vi "绑定设备.vi"(8 "error in (no error)":errorcluster, 10 "设备注册-来自PC总客户端":T1, 11 "数据库操作.i":refnum<class "数据库操作.lvclass">) -> (0 "error out":errorcluster, 3 "数据库操作.o":refnum<class "数据库操作.lvclass">)   [LabVIEW 2013, in "数据库操作.lvclass"]
uses:
  <vilib>/addons/database/Connection.llb/Conn Execute.vi
  <vilib>/addons/database/NI_Database_API.lvlib
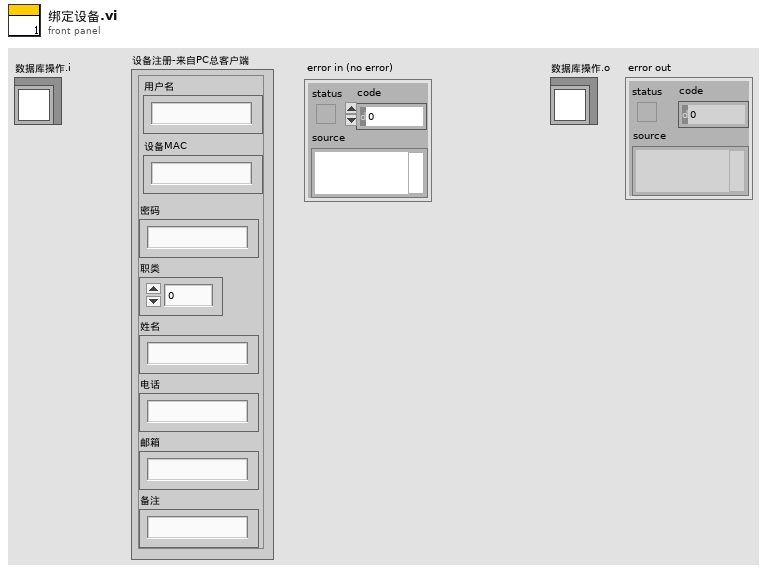
[diagram p1: front panel]
types:
  T1 = cluster{"设备MAC":string, "密码":string, "职类":i32, "姓名":string, "电话":string, "邮箱":string, "备注":string, "用户名":string}
  T2 = typedef "NI_Database_API.lvlib/Conn ObjectReference.ctl" = refnum<k1>
  T3 = cluster{"用户名":string, "设备状态":i32, "密码":string, "职类":i32, "姓名":string, "电话":string, "邮箱":string, "备注":string, "最后活动":string}
  T4 = enum16{"用户名", "设备MAC", "设备状态", "密码", "职类", "姓名", "电话", "邮箱", "备注", "最后活动"}
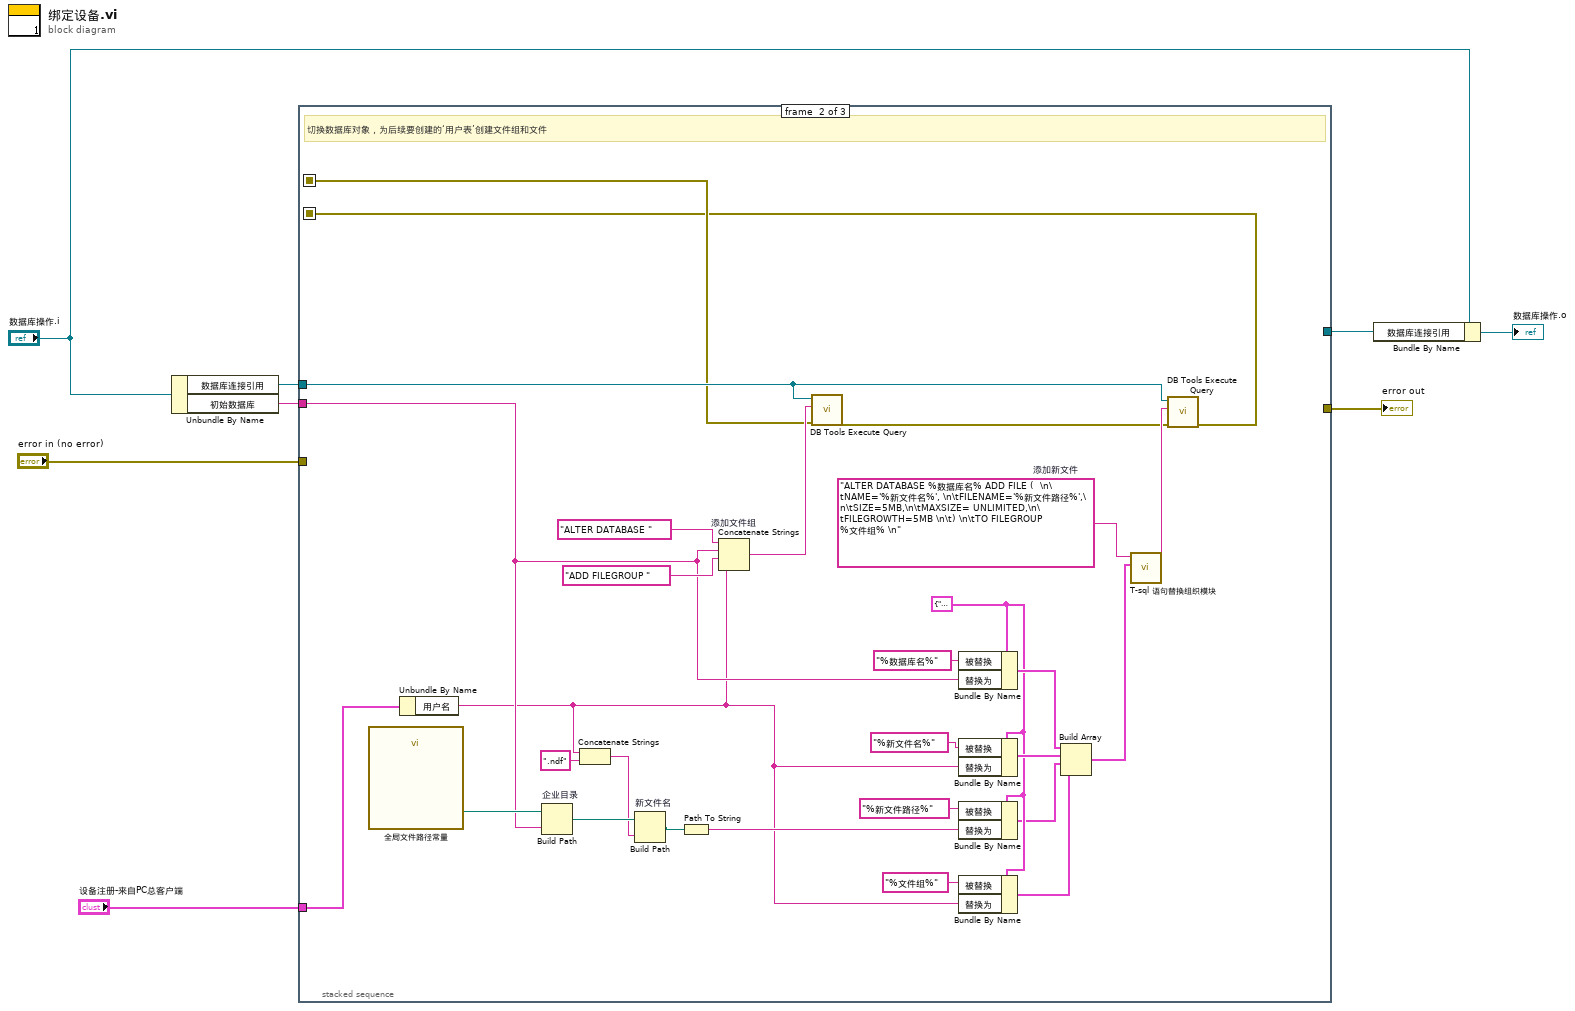
[diagram p0: block diagram]
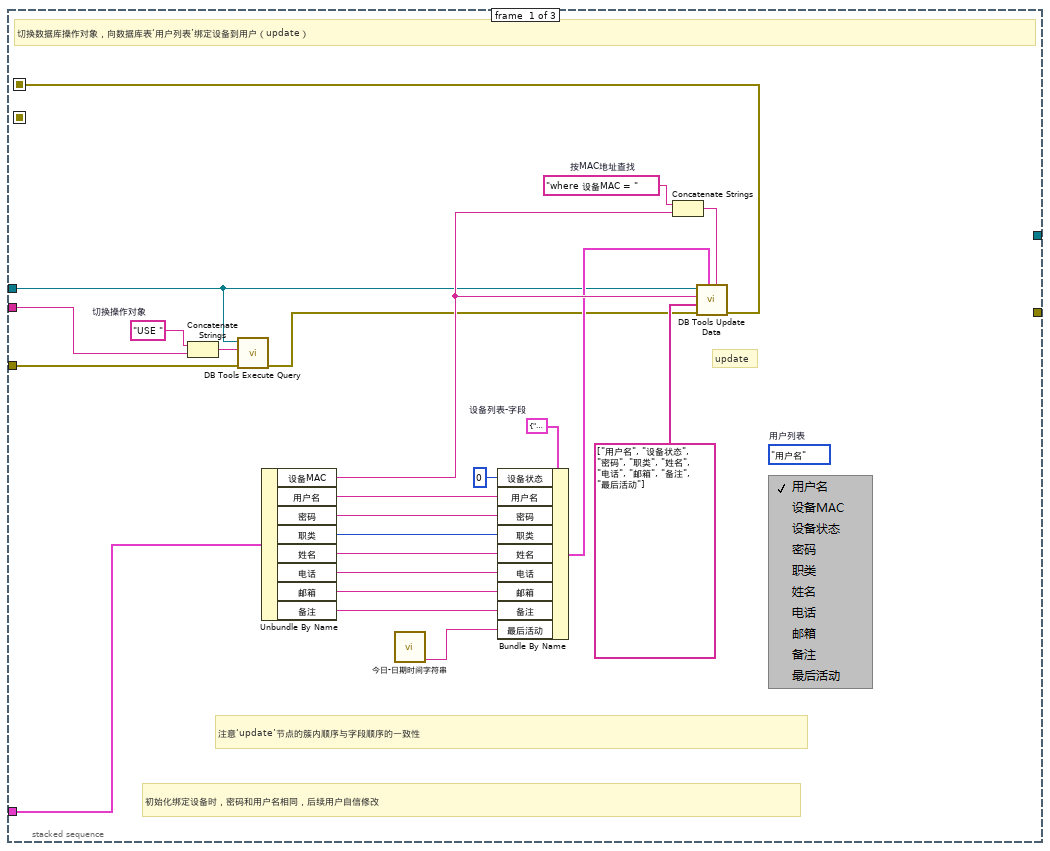
[diagram p2: hidden frame]
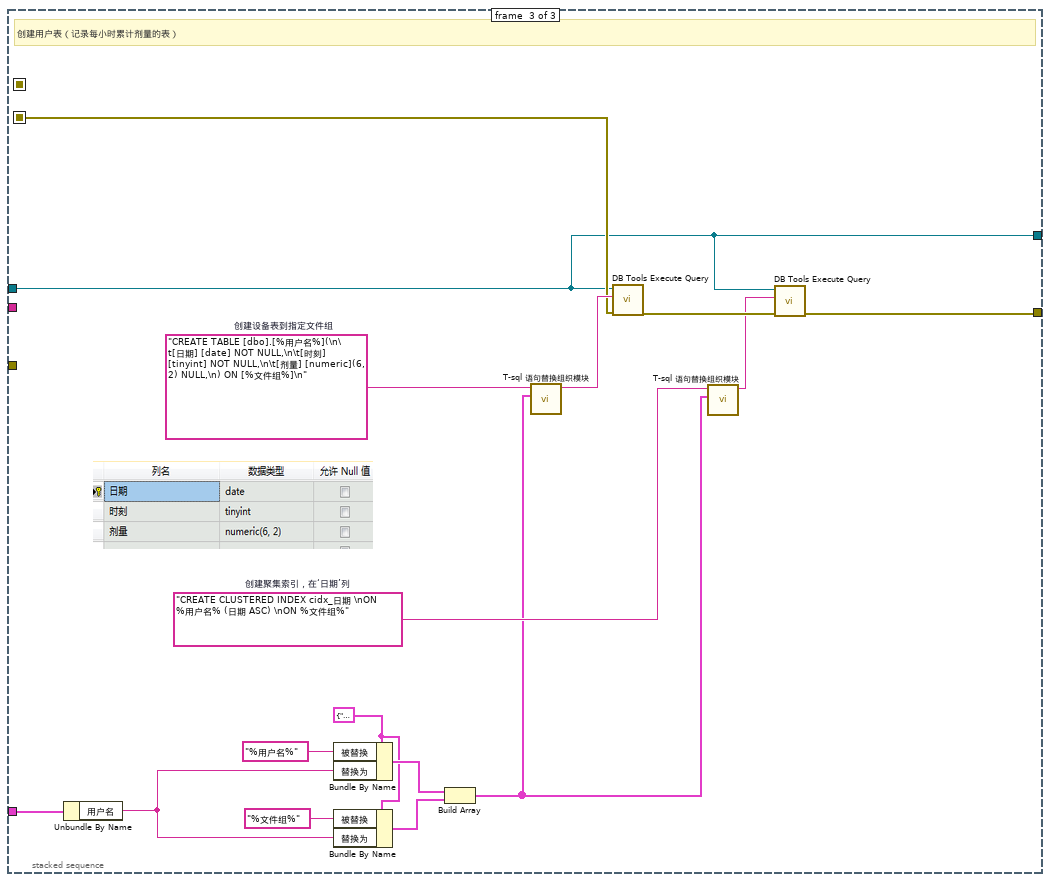
[diagram p3: hidden frame]
diagram:
  n1 = Unbundle By Name("数据库操作.i") -> ("数据库连接引用"=w6:T2, "初始数据库"=w8:string)
  n2 = stacked-sequence {
    seq-local: [w10 _ _] -> [_ w33 _]
    seq-local: [_ w32 _] -> [_ _ w66]
    tunnel: w8 -> [w14 w51 _]
    tunnel: w6 -> [w9 w36 w63]
    tunnel: "设备注册-来自PC总客户端" -> [w16 w35 w68]
    tunnel: "error in (no error)" -> [w12 _ _]
    tunnel: [_ _ w64] -> w4
    tunnel: [_ _ w63] -> w3
    frame #0 {
      w15 = "USE "  # 切换操作对象
      w29 = "where 设备MAC = "  # 按MAC地址查找
      w17 = T3 {"用户名"="", "设备状态"=0, "密码"="", "职类"=0, "姓名"="", "电话"="", "邮箱"="", "备注"="", "最后活动"=""}  # 设备列表-字段
      (unwired) T4."用户名"  # 用户列表
      # "初始化绑定设备时，密码和用户名相同，后续用户自信修改"
      # "注意‘update’节点的簇内顺序与字段顺序的一致性"
      # "update"
      # "切换数据库操作对象，向数据库表‘用户列表’绑定设备到用户（update）"
      n3 = Concatenate Strings(w15, w14) -> (w13:string)
      n4 = call-poly <vilib>:"DB Tools Execute Query.vi"("error in (no error)"=w12, "SQL query"=w13, "connection reference"=w9) -> ("error out"=w11:errorcluster)  [unwired: 5 in, 1 out]
      n5 = Unbundle By Name(w16) -> ("设备MAC"=w30:string, "用户名"=w18:string, "密码"=w19:string, "职类"=w20:i32, "姓名"=w21:string, "电话"=w22:string, "邮箱"=w23:string, "备注"=w24:string)
      n6 = call "今日-日期时间字符串.vi"() -> ("日期时间"=w28:string)  [unwired: 9 in, 2 out]
      n7 = Bundle By Name(cluster=w17, "设备状态"=0, "用户名"=w18, "密码"=w19, "职类"=w20, "姓名"=w21, "电话"=w22, "邮箱"=w23, "备注"=w24, "最后活动"=w28) -> (w25:T3)
      n8 = Concatenate Strings(w29, w30) -> (w31:string)
      n9 = call <vilib>:"DB Tools Update Data.vi"("condition"=w31, "data"=w25, "error in (no error)"=w11, "columns"=string[] ["用户名", "设备状态", "密码", "职类", "姓名", "电话", "邮箱", "备注", "最后活动"], "table"=w30, "connection reference"=w9) -> ("error out"=w10:errorcluster)  [unwired: 4 in, 1 out]
    }
    frame #1 {
      w39 = "ALTER DATABASE %数据库名% ADD FILE (  \n\tNAME='%新文件名%', \n\tFILENAME='%新文件路径%',\n\tSIZE=5MB,\n\tMAXSIZE= UNLIMITED,\n\tFILEGROWTH=5MB \n\t) \n\tTO FILEGROUP %文件组% \n"  # 添加新文件
      w43 = cluster{"被替换":string, "替换为":string} {"被替换"="", "替换为"=""} ("替换单元")
      # "切换数据库对象，为后续要创建的‘用户表’创建文件组和文件"
      n10 = call "全局文件路径常量.vi"() -> ("用户数据库根目录"=w52:path)  [unwired: 9 in, 2 out]
      n11 = Unbundle By Name(w35) -> ("用户名"=w34:string)
      n12 = Build Path "企业目录"(base path=w52, name or relative path=w51) -> (appended path=w50:path)
      n13 = Concatenate Strings(w34, ".ndf" ("字符串")) -> (w48:string)
      n14 = Build Path "新文件名"(base path=w50, name or relative path=w48) -> (appended path=w47:path)
      n15 = Path To String(path=w47) -> (string=w46:string)
      n16 = Concatenate Strings "添加文件组"("ALTER DATABASE " ("SQL query"), w51, "ADD FILEGROUP " ("SQL query"), w34) -> (w57:string)
      n17 = call-poly <vilib>:"DB Tools Execute Query.vi"("error in (no error)"=w33, "SQL query"=w57, "connection reference"=w36) -> ("error out"=w37:errorcluster)  [unwired: 5 in, 1 out]
      n18 = Bundle By Name(cluster=w43, "被替换"="%数据库名%", "替换为"=w51) -> (w45:cluster{"被替换":string, "替换为":string})
      n19 = Bundle By Name(cluster=w43, "被替换"="%新文件名%", "替换为"=w34) -> (w44:cluster{"被替换":string, "替换为":string})
      n20 = Bundle By Name(cluster=w43, "被替换"="%新文件路径%", "替换为"=w46) -> (w42:cluster{"被替换":string, "替换为":string})
      n21 = Bundle By Name(cluster=w43, "被替换"="%文件组%", "替换为"=w34) -> (w41:cluster{"被替换":string, "替换为":string})
      n22 = Build Array(w45, w44, w42, w41) -> (w40:cluster{"被替换":string, "替换为":string}[])
      n23 = call "T-sql 语句替换组织模块.vi"("替换项"=w40, "T-sql 模板"=w39) -> ("T-sql"=w38:string)  [unwired: 8 in, 1 out]
      n24 = call-poly <vilib>:"DB Tools Execute Query.vi"("error in (no error)"=w37, "SQL query"=w38, "connection reference"=w36) -> ("error out"=w32:errorcluster)  [unwired: 5 in, 1 out]
    }
    frame #2 {
      w62 = "CREATE CLUSTERED INDEX cidx_日期 \nON %用户名% (日期 ASC) \nON %文件组%"  # 创建聚集索引，在‘日期’列
      w69 = cluster{"被替换":string, "替换为":string} {"被替换"="", "替换为"=""} ("替换单元")
      w74 = "CREATE TABLE [dbo].[%用户名%](\n\t[日期] [date] NOT NULL,\n\t[时刻] [tinyint] NOT NULL,\n\t[剂量] [numeric](6, 2) NULL,\n) ON [%文件组%]\n"  # 创建设备表到指定文件组
      # "创建用户表（记录每小时累计剂量的表）"
      n25 = Unbundle By Name(w68) -> ("用户名"=w67:string)
      n26 = Bundle By Name(cluster=w69, "被替换"="%用户名%", "替换为"=w67) -> (w72:cluster{"被替换":string, "替换为":string})
      n27 = Bundle By Name(cluster=w69, "被替换"="%文件组%", "替换为"=w67) -> (w73:cluster{"被替换":string, "替换为":string})
      n28 = Build Array(w72, w73) -> (w61:cluster{"被替换":string, "替换为":string}[])
      n29 = call "T-sql 语句替换组织模块.vi"("替换项"=w61, "T-sql 模板"=w74) -> ("T-sql"=w75:string)  [unwired: 8 in, 1 out]
      n30 = call-poly <vilib>:"DB Tools Execute Query.vi"("error in (no error)"=w66, "SQL query"=w75, "connection reference"=w63) -> ("error out"=w65:errorcluster)  [unwired: 5 in, 1 out]
      n31 = call "T-sql 语句替换组织模块.vi"("替换项"=w61, "T-sql 模板"=w62) -> ("T-sql"=w60:string)  [unwired: 8 in, 1 out]
      n32 = call-poly <vilib>:"DB Tools Execute Query.vi"("error in (no error)"=w65, "SQL query"=w60, "connection reference"=w63) -> ("error out"=w64:errorcluster)  [unwired: 5 in, 1 out]
    }
  }
  "error out" <- w4
  n33 = Bundle By Name(cluster="数据库操作.i", "数据库连接引用"=w3) -> (→"数据库操作.o":refnum<class "数据库操作.lvclass">)
